vi "Configure Sequence (Staircase).vi"(0 "VISA resource name":refnum<visa-resource-name>, 1 "Channel Name (1)":string="1", 3 "Staircase Sequence Steps (10)":i32=10, 4 "Waveform Type (1: Voltage)":i32(ring)=1 items=["Voltage"=1, "Current"=0], 5 "error in (no error)":errorcluster {"code" format="%.0x"}, 6 "Staircase Sequence Start Time (0.0 s)":dbl format="%^.3e", 7 "Staircase Sequence End Time (0.0 s)":dbl format="%^.3e", 8 "Staircase Sequence Start Level (0.0)":dbl format="%^.3e", 9 "Staircase Sequence End Level (0.0)":dbl format="%^.3e", 10 "Staircase Sequence Total Time (1.0 s)":dbl=1.0 format="%^.3e", 12 "Sequence Step Number (0)":i32) -> (14 "VISA resource name out":refnum<visa-resource-name>, 19 "error out":errorcluster {"code" format="%.0x"})   [LabVIEW 2016, in "Agilent N6700 Series.lvlib"]
doc: "Configures the staircase sequence.\n\n<b>Note:</b>\nThis VI only applies to the N6705B and N6705C DC Power Analyzer."
uses:
  <instrlib>/Agilent N6700 Series/Agilent N6700 Series.lvlib
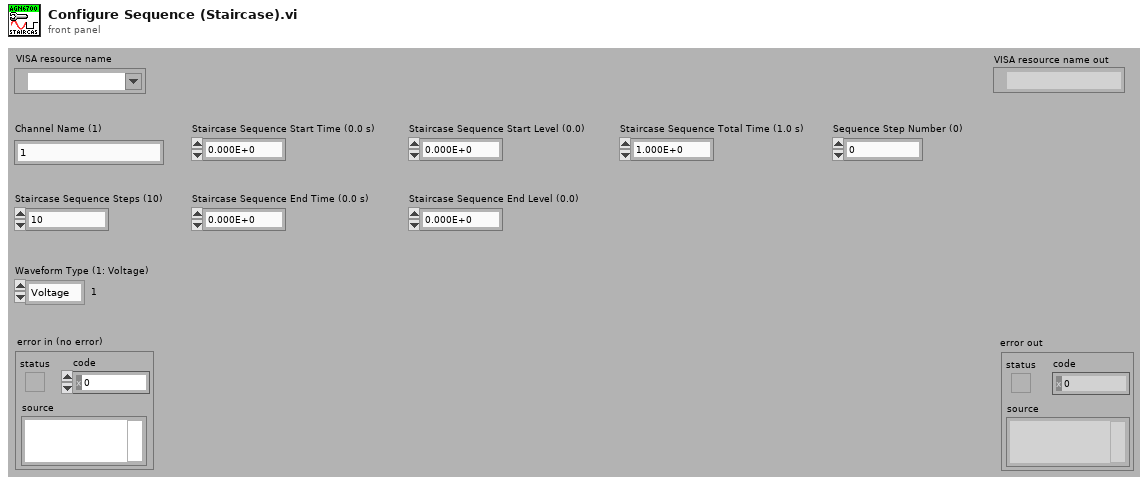
[diagram p1: front panel]
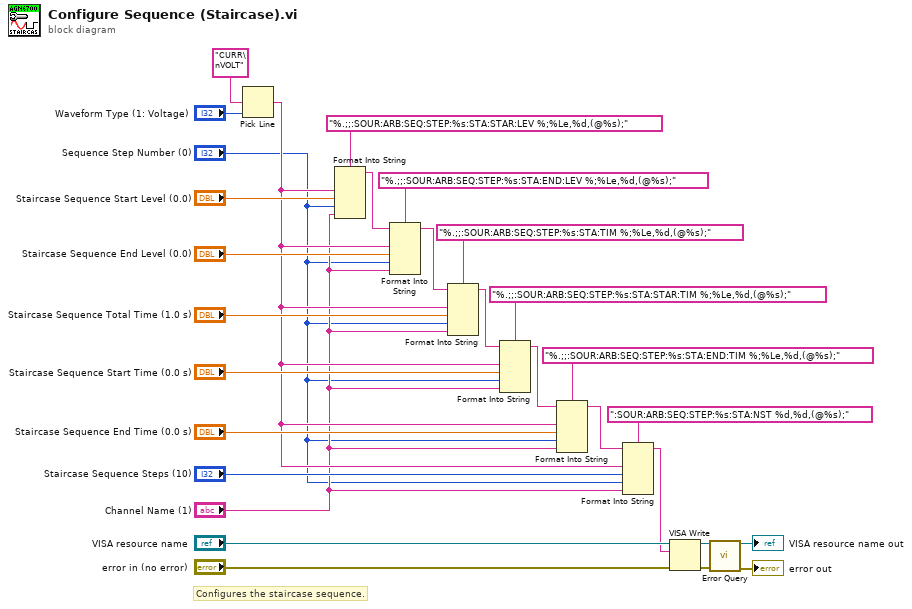
[diagram p0: block diagram]
diagram:
  # "Configures the staircase sequence."
  n1 = Pick Line(multi-line string="CURR\nVOLT", line index="Waveform Type (1: Voltage)") -> (output string=w3:string)  [unwired: 1 in]
  n2 = Format Into String(format string="%.;;:SOUR:ARB:SEQ:STEP:%s:STA:STAR:LEV %;%Le,%d,(@%s);", w3, "Staircase Sequence Start Level (0.0)", "Sequence Step Number (0)", "Channel Name (1)") -> (resulting string=w19:string)  [unwired: 2 in, 1 out]
  n3 = Format Into String(format string="%.;;:SOUR:ARB:SEQ:STEP:%s:STA:END:LEV %;%Le,%d,(@%s);", initial string=w19, w3, "Staircase Sequence End Level (0.0)", "Sequence Step Number (0)", "Channel Name (1)") -> (resulting string=w18:string)  [unwired: 1 in, 1 out]
  n4 = Format Into String(format string="%.;;:SOUR:ARB:SEQ:STEP:%s:STA:TIM %;%Le,%d,(@%s);", initial string=w18, w3, "Staircase Sequence Total Time (1.0 s)", "Sequence Step Number (0)", "Channel Name (1)") -> (resulting string=w17:string)  [unwired: 1 in, 1 out]
  n5 = Format Into String(format string="%.;;:SOUR:ARB:SEQ:STEP:%s:STA:STAR:TIM %;%Le,%d,(@%s);", initial string=w17, w3, "Staircase Sequence Start Time (0.0 s)", "Sequence Step Number (0)", "Channel Name (1)") -> (resulting string=w16:string)  [unwired: 1 in, 1 out]
  n6 = Format Into String(format string="%.;;:SOUR:ARB:SEQ:STEP:%s:STA:END:TIM %;%Le,%d,(@%s);", initial string=w16, w3, "Staircase Sequence End Time (0.0 s)", "Sequence Step Number (0)", "Channel Name (1)") -> (resulting string=w6:string)  [unwired: 1 in, 1 out]
  n7 = Format Into String(format string=":SOUR:ARB:SEQ:STEP:%s:STA:NST %d,%d,(@%s);", initial string=w6, w3, "Staircase Sequence Steps (10)", "Sequence Step Number (0)", "Channel Name (1)") -> (resulting string=w4:string)  [unwired: 1 in, 1 out]
  n8 = VISA Write(VISA resource name="VISA resource name", write buffer=w4, error in (no error)="error in (no error)") -> (VISA resource name out=w25:refnum<visa-resource-name>, error out=w24:errorcluster)  [unwired: 1 out]
  n9 = call <instrlib>:"Error Query.vi"("VISA resource name"=w25, "error in (no error)"=w24) -> ("VISA resource name out"=→"VISA resource name out":refnum<visa-resource-name>, "error out"=→"error out":errorcluster)  [unwired: 10 in, 2 out]
